vi "Extract data from string.vi"(8 "error in (no error)":errorcluster, 9 "End of data":string, 10 "Start of data":string, 11 "string in":string) -> (0 "error out":errorcluster, 3 "Extracted data":string)   [LabVIEW 2013]
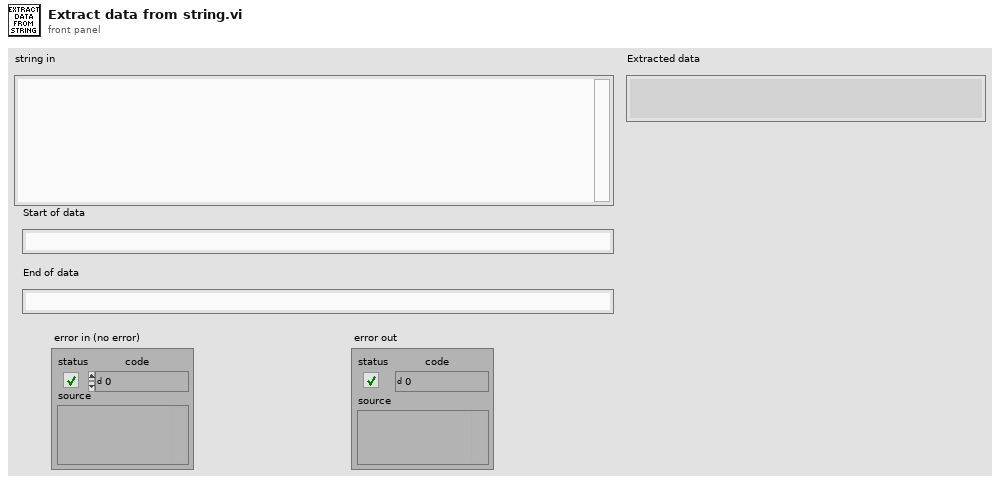
[diagram p1: front panel]
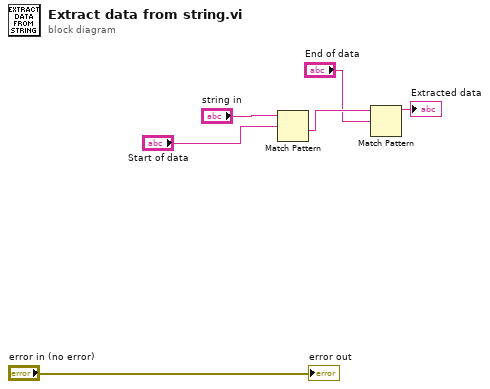
[diagram p0: block diagram]
diagram:
  n1 = Match Pattern(string="string in", regular expression="Start of data") -> (after substring=w4:string)  [unwired: 1 in, 3 out]
  n2 = Match Pattern(string=w4, regular expression="End of data") -> (before substring=→"Extracted data":string)  [unwired: 1 in, 3 out]
  "error out" <- "error in (no error)"
